vi "Queue Up Inital Action.vi"(8 "Error In":errorcluster, 11 "List of Initalisation commands":string[](array[string])=["FrontPanel FullScreen", "FrontPanel ScaleSideTab", "FrontPanel LoadUserConfiguration", "Mapping Initalise", "Mapping ResetWaypoints", "Mapping LoadEvents", "Vision ConnectToCamera"]) -> (0 "Error Out":errorcluster)   [LabVIEW 2014]
uses:
  Data Processing Queue/SubVI/Set Multiple Operations.vi
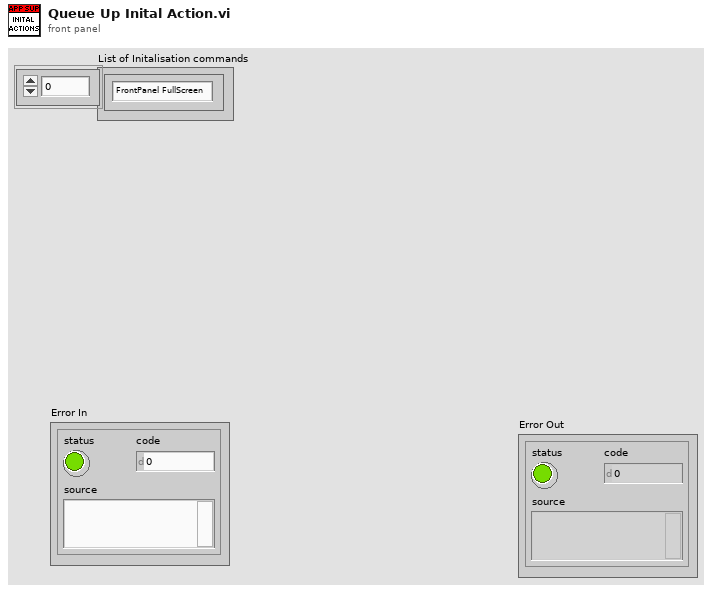
[diagram p1: front panel]
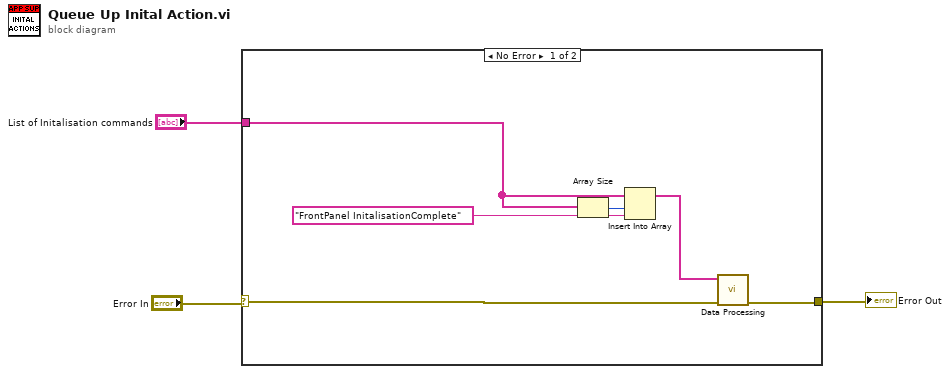
[diagram p0: block diagram]
diagram:
  n1 = case shown="No Error" "Error In" {
    selector: "Error In" -> [w6 w10]
    tunnel: "List of Initalisation commands" -> [w7 _]
    tunnel: [w5 w10] -> w1
    frame No Error {
      n2 = Array Size(array=w7) -> (size(s)=w8:i32)
      n3 = Insert Into Array(array=w7, index=w8, new element="FrontPanel InitalisationComplete" ("Command")) -> (w4:string[])
      n4 = call-poly "Data Processing.vi"("error in (no error)"=w6, "Command"=w4) -> ("error out"=w5:errorcluster)  [unwired: 9 in]
    }
    frame Error {
    }
  }
  "Error Out" <- w1
